vi "Get Entity Paths OoC.vi"(11 "Entity Path":path) -> (3 "Entity Paths":T1)   [LabVIEW 2020, in "Conditum-Tools.lvlib" / "Entity Editor.lvclass"]
uses:
  Entity Editor.lvclass
  Entity Paths.ctl
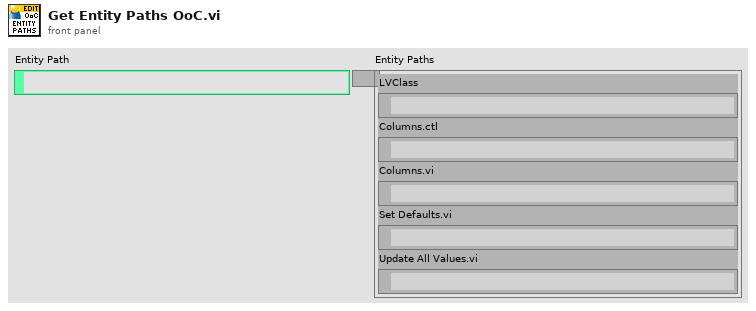
[diagram p1: front panel]
types:
  T1 = typedef "Conditum-Tools.lvlib/Entity Editor.lvclass/Entity Paths.ctl" = cluster{"LVClass":path, "Columns.ctl":path, "Columns.vi":path, "Set Defaults.vi":path, "Update All Values.vi":path}
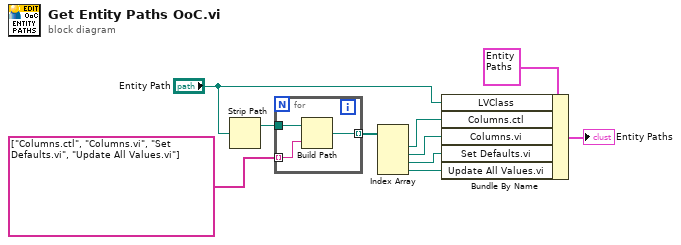
[diagram p0: block diagram]
diagram:
  n1 = Strip Path(path="Entity Path") -> (stripped path=w8:path)  [unwired: 1 out]
  n2 = for {
    tunnel: string[] ["Columns.ctl", "Columns.vi", "Set Defaults.vi", "Update All Values.vi"] -> [w11] mode=indexing
    tunnel: w8 -> [w12]
    tunnel: [w13] -> w9 mode=indexing
    n3 = Build Path(base path=w12, name or relative path=w11) -> (appended path=w13:path)
  }
  n4 = Index Array(array=w9) -> (element #1=w2:path, element #2=w3:path, element #3=w4:path, element #4=w5:path)  [unwired: 4 in]
  n5 = Bundle By Name(cluster=T1 {"LVClass"=path "", "Columns.ctl"=path "", "Columns.vi"=path "", "Set Defaults.vi"=path "", "Update All Values.vi"=path ""} ("Entity Paths"), "LVClass"="Entity Path", "Columns.ctl"=w2, "Columns.vi"=w3, "Set Defaults.vi"=w4, "Update All Values.vi"=w5) -> (→"Entity Paths":T1)
